vi "dsf shared data dvr property name.vi"() -> (3 "shared data dvr property name":string)   [LabVIEW 2020, in "DSF Shared.lvlib"]
uses:
  DSF Shared.lvlib
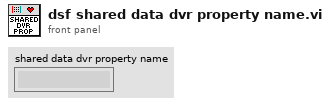
[diagram p1: front panel]
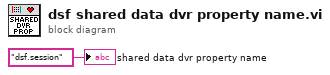
[diagram p0: block diagram]
diagram:
  "shared data dvr property name" <- "dsf.session" ("Property Name")
